vi "Read_file.vi"() -> ()   [LabVIEW 2011]
panel:
  out "XY Graph 2":cluster{"Y":dbl[], "Y":dbl[]}[](graph)
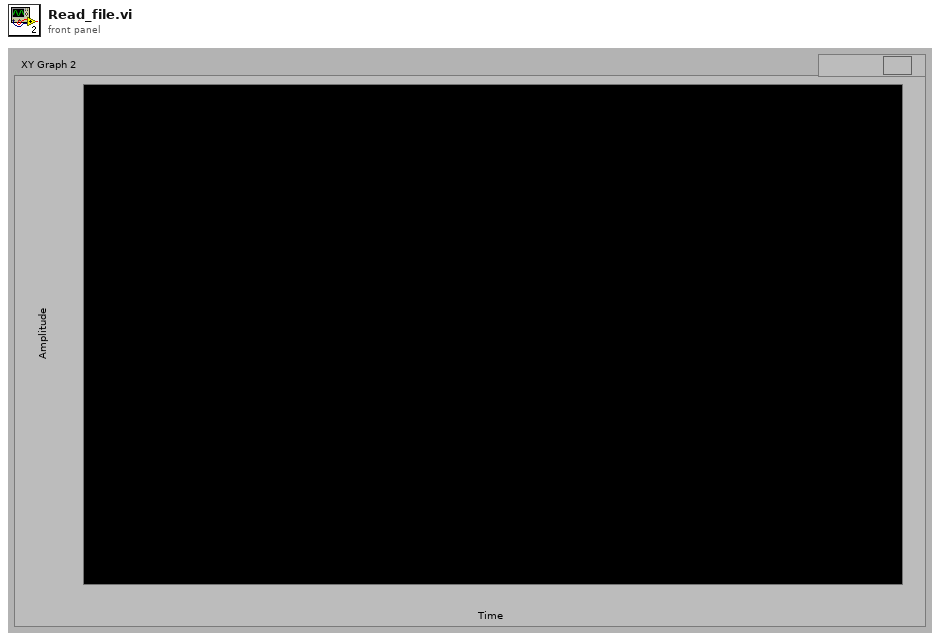
[diagram p1: front panel]
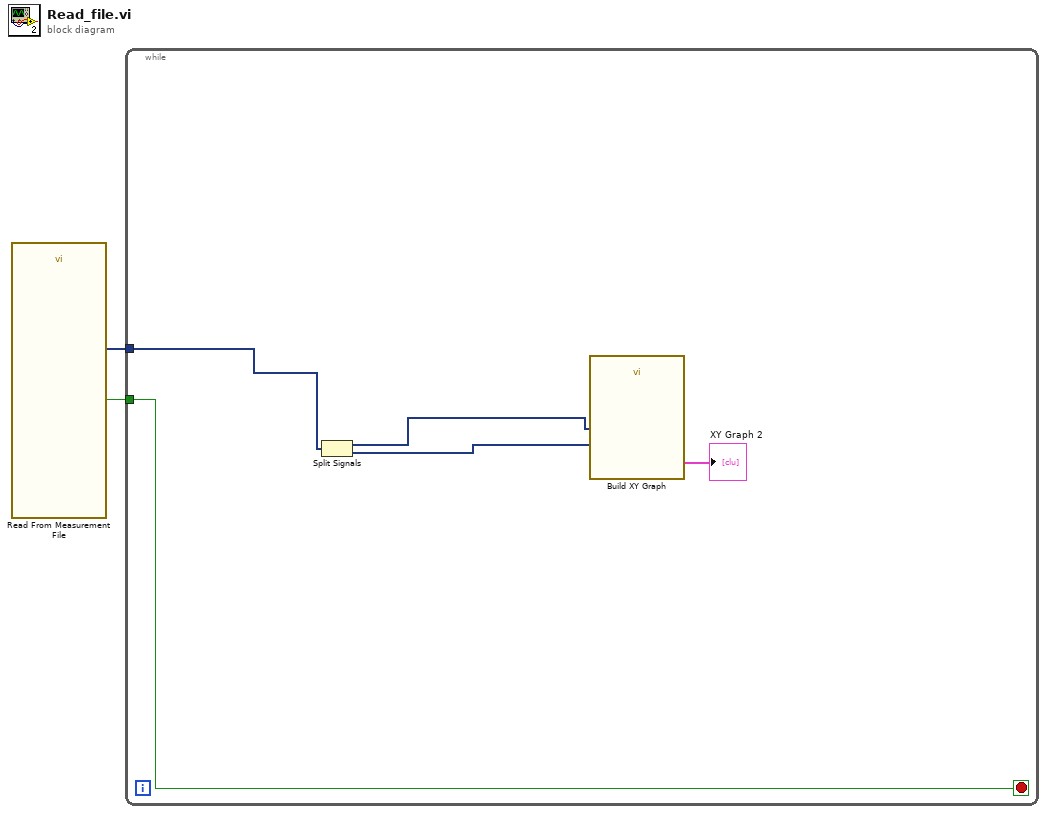
[diagram p0: block diagram]
diagram:
  n1 = call "Read From Measurement File"() -> ("Signals"=w2:dynamicdata, "EOF?"=w1:bool)  [unwired: 6 in, 4 out]
  n2 = while {
    tunnel: w2 -> [w7]
    tunnel: w1 -> [w6]
    stop <- w6 stop-if-true
    n3 = Split Signals(w7) -> (w4:dynamicdata, w3:dynamicdata)  [unwired: 2 in]
    n4 = call "Build XY Graph"("Y Input"=w3, "X Input"=w4) -> ("XY Graph"=→"XY Graph 2":cluster{"Y":dbl[], "Y":dbl[]}[])  [unwired: 3 in, 6 out]
  }
